vi "Configure Calibration Factor Table.vi"(4 "Frequency Array (0.0)":dbl[](array[numeric]), 6 "Calibration Factor Array (0.0)":dbl[](array[numeric]), 8 "error in (no error)":errorcluster, 9 "Array Size (0)":i32, 10 "Power Sensor (0: Power Sensor A)":u16(ring) items=["Power Sensor A", "Power Sensor B"], 11 "VISA resource name":refnum<visa-resource-name>) -> (0 "error out":errorcluster, 3 "VISA resource name out":refnum<visa-resource-name>)   [LabVIEW 2018, in "Agilent ENA Series.lvlib"]
doc: "Sets the calibration factor table for selected power sensor."
uses:
  Agilent ENA Series.lvlib
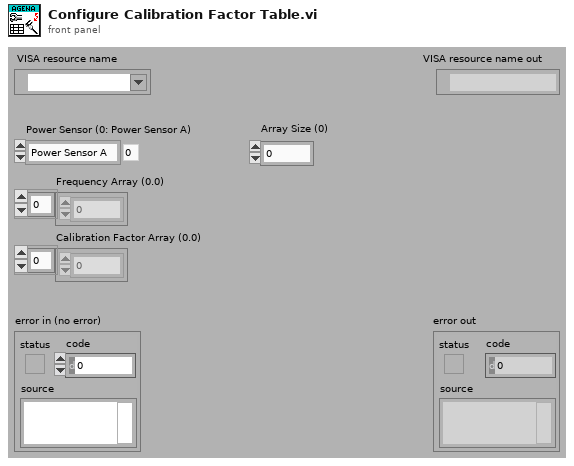
[diagram p1: front panel]
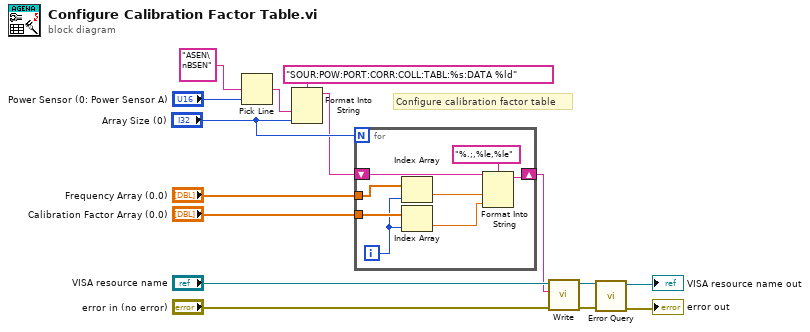
[diagram p0: block diagram]
diagram:
  # "Configure calibration factor table"
  n1 = Pick Line(multi-line string="ASEN\nBSEN", line index="Power Sensor (0: Power Sensor A)") -> (output string=w11:string)  [unwired: 1 in]
  n2 = Format Into String(format string="SOUR:POW:PORT:CORR:COLL:TABL:%s:DATA %ld", w11, "Array Size (0)") -> (resulting string=w6:string)  [unwired: 2 in, 1 out]
  n3 = for {
    N: "Array Size (0)" -> [_]
    tunnel: "Frequency Array (0.0)" -> [w18]
    tunnel: "Calibration Factor Array (0.0)" -> [w20]
    shift-right: [w21] -> w5
    shift-left: w6 -> [w23]
    i -> [w17]
    n4 = Index Array(array=w18, index=w17) -> (element=w16:dbl)
    n5 = Index Array(array=w20, index=w17) -> (element=w19:dbl)
    n6 = Format Into String(format string="%.;,%le,%le", initial string=w23, w16, w19) -> (resulting string=w21:string)  [unwired: 1 in, 1 out]
  }
  n7 = call "Write.vi"("error in (no error)"="error in (no error)", "String ()"=w5, "VISA resource name"="VISA resource name") -> ("error out"=w3:errorcluster, "VISA resource name out"=w4:refnum<visa-resource-name>)  [unwired: 6 in, 1 out]
  n8 = call "Error Query.vi"("error in (no error)"=w3, "VISA resource name"=w4) -> ("error out"=→"error out":errorcluster, "VISA resource name out"=→"VISA resource name out":refnum<visa-resource-name>)  [unwired: 6 in, 2 out]
